vi "armBackDownCode.vi"() -> (2 "armMotorValue":dbl, 3 "intakePneumaticValue":bool)   [LabVIEW 2013]
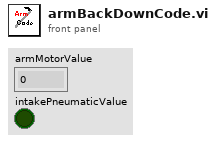
[diagram p1: front panel]
types:
  T1 = typedef "WPI_EncoderDevRef.ctl" = cluster{"DevStatus":errorcluster, "EncoderIndex":T2, "CounterIndex":T3, "DistancePerCount":dbl, "Decoding Type":T4}
  T2 = typedef "FPGA_EncoderIdx.ctl" = enum8{"Enc 0", "Enc 1", "Enc 2", "Enc 3", "Invalid"}
  T3 = typedef "FPGA_CounterCtrSystemIndex.ctl" = enum8{"Ctr 0", "Ctr 1", "Ctr 2", "Ctr 3", "Ctr 4", "Ctr 5", "Ctr 6", "Ctr 7", "Invalid"}
  T4 = typedef "WPI_EncoderType.ctl" = enum16{"1x", "2x", "4x"}
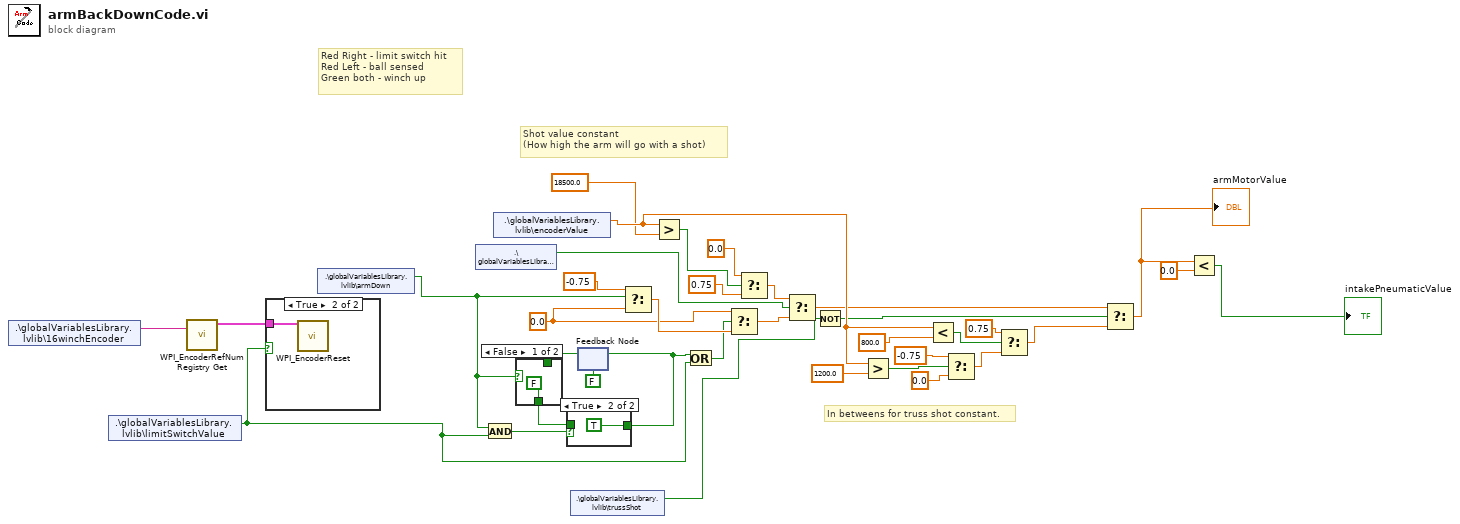
[diagram p0: block diagram]
diagram:
  w7 = 0.0 ("f")
  # "Red Right - limit switch hit\nRed Left - ball sensed\nGreen both - winch up"
  # "In betweens for truss shot constant."
  # "Shot value constant\n(How high the arm will go with a shot)"
  n1 = shared-variable ".\\globalVariablesLibrary.lvlib\\16winchEncoder"() -> (w15:string)  [unwired: 1 in, 1 out]
  n2 = shared-variable ".\\globalVariablesLibrary.lvlib\\limitSwitchValue"() -> (w17:bool)  [unwired: 1 in, 1 out]
  n3 = call <vilib>:"WPI_EncoderRefNum Registry Get.vi"("refnum name"=w15) -> ("EncoderDevRef"=w16:T1)  [unwired: 9 in, 1 out]
  n4 = case shown="True" w17 {
    tunnel: w16 -> [_ w37]
    frame False {
    }
    frame True {
      n5 = call <vilib>:"WPI_EncoderReset.vi"("EncoderDevRef"=w37) -> ()  [unwired: 9 in, 2 out]
    }
  }
  n6 = shared-variable ".\\globalVariablesLibrary.lvlib\\armDown"() -> (w33:bool)  [unwired: 1 in, 1 out]
  n7 = shared-variable ".\\globalVariablesLibrary.lvlib\\armUp"() -> (w35:bool)  [unwired: 1 in, 1 out]
  n8 = And(x=w33, y=w17) -> (x .and. y?=w6:bool)
  n9 = shared-variable ".\\globalVariablesLibrary.lvlib\\encoderValue"() -> (w30:dbl)  [unwired: 1 in, 1 out]
  n10 = shared-variable ".\\globalVariablesLibrary.lvlib\\trussShot"() -> (w34:bool)  [unwired: 1 in, 1 out]
  n11 = feedback #1(FALSE) -> (w3:bool)
  n12 = case shown="False" w33 {
    tunnel: [FALSE w39] -> w4
    tunnel: w3 -> [_ w39]
    frame False {
    }
    frame True {
    }
  }
  n13 = case shown="True" w6 {
    tunnel: [w40 TRUE] -> w1
    tunnel: w4 -> [w40 _]
    frame False {
    }
    frame True {
    }
  }
  n14 = feedback-in #1(w1) -> ()
  n15 = Select(t=-0.75, s=w33, f=w7) -> (s? t:f=w9:dbl)
  n16 = Greater?(x=w30, y=18500.0) -> (0:w13:bool)
  n17 = Or(x=w1, y=w17) -> (x .or. y?=w2:bool)
  n18 = Select(t=w7, s=w2, f=w9) -> (s? t:f=w8:dbl)
  n19 = Select(t=0.0, s=w13, f=0.75) -> (s? t:f=w11:dbl)
  n20 = Select(t=w11, s=w35, f=w8) -> (s? t:f=w18:dbl)
  n21 = Not(x=w34) -> (.not. x?=w19:bool)
  n22 = Greater?(x=w30, y=1200.0) -> (0:w26:bool)
  n23 = Less?(x=w30, y=800.0) -> (x < y?=w22:bool)
  n24 = Select(t=-0.75, s=w26, f=0.0) -> (s? t:f=w24:dbl)
  n25 = Select(t=0.75, s=w22, f=w24) -> (s? t:f=w28:dbl)
  n26 = Select(t=w18, s=w19, f=w28) -> (s? t:f=w31:dbl)
  "armMotorValue" <- w31
  n27 = Less?(x=w31, y=0.0) -> (x < y?=→"intakePneumaticValue":bool)
